vi "Target Resistance.vi"(0 "instrument handle":refnum<k15>="PXI1Slot2 (869)", 1 "Max attempts":dbl=10.0 format="%#_13g", 5 "Lower resistance (ohm)":dbl=80000.0, 9 "Upper resistance (ohm)":dbl=100000.0, 11 "error in (no error)":errorcluster) -> (3 "SL voltage (V)":dbl=2.6, 4 "instrument handle out":refnum<k15>="PXI1Slot2 (869)", 6 "final resistance (ohm)":dbl format="%#_6p", 8 "target hit?":bool, 10 "final current (A)":dbl, 12 "BL voltage (V)":dbl=2.6, 14 "WL voltage (V)":dbl=1.7, 15 "error out":errorcluster)   [LabVIEW 2018]
panel:
  out "attempt number":i32=15
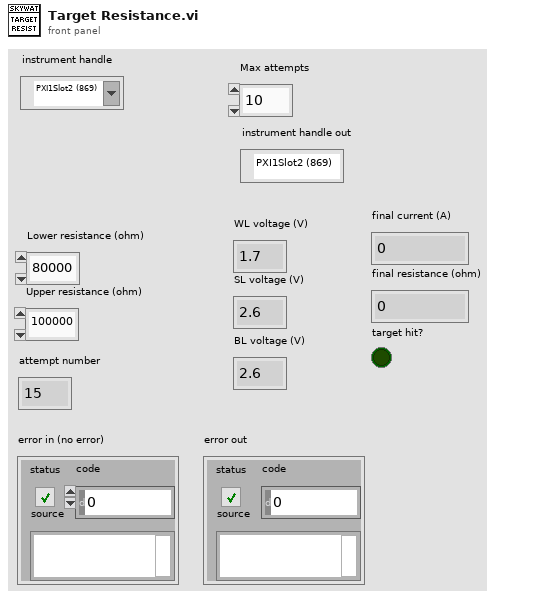
[diagram p1: front panel]
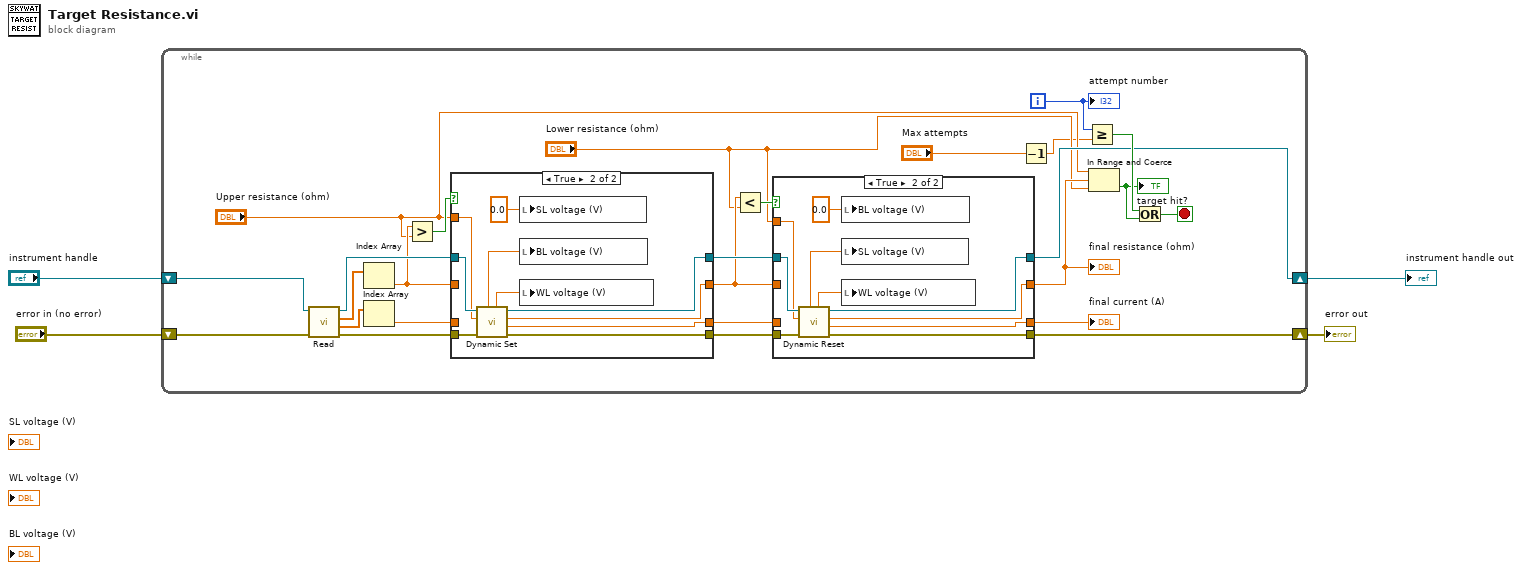
[diagram p0: block diagram]
diagram:
  n1 = while {
    shift-right: [w18] -> w3
    shift-left: "instrument handle" -> [w30]
    shift-right: [w17] -> w2
    shift-left: "error in (no error)" -> [w29]
    i -> [w23]
    stop <- w24 stop-if-true
    n2 = call "Read.vi"("error in (no error)"=w29, "instrument handle"=w30) -> ("error out"=w25:errorcluster, "currents (A)"=w15:dbl[], "resistances (ohm)"=w28:dbl[], "instrument handle out"=w26:refnum<k15>)  [unwired: 6 in]
    n3 = Index Array(array=w28) -> (element=w16:dbl)  [unwired: 1 in]
    n4 = Index Array(array=w15) -> (element=w14:dbl)  [unwired: 1 in]
    n5 = Greater?(x=w16, y="Upper resistance (ohm)") -> (0:w27:bool)
    n6 = case shown="True" w27 {
      tunnel: w26 -> [w48 w56]
      tunnel: w25 -> [w47 w55]
      tunnel: [w48 w57] -> w20
      tunnel: [w47 w58] -> w19
      tunnel: [w46 w54] -> w8
      tunnel: w16 -> [w46 _]
      tunnel: w14 -> [w45 _]
      tunnel: [w45 w53] -> w13
      tunnel: "Upper resistance (ohm)" -> [_ w49]
      frame False {
      }
      frame True {
        n7 = call "Dynamic Set.vi"("error in (no error)"=w55, "target resistance (ohm)"=w49, "instrument handle"=w56) -> ("error out"=w58:errorcluster, "final current (A)"=w53:dbl, "final resistance (ohm)"=w54:dbl, "instrument handle out"=w57:refnum<k15>, "WL voltage (V)"=w52:dbl, "BL voltage (V)"=w51:dbl)  [unwired: 2 in, 1 out]
        n8 = local write "SL voltage (V)"(0.0 ("SL voltage (V)")) -> ()
        n9 = local write "BL voltage (V)"(w51) -> ()
        n10 = local write "WL voltage (V)"(w52) -> ()
      }
    }
    n11 = Less?(x=w8, y="Lower resistance (ohm)") -> (x < y?=w9:bool)
    n12 = case shown="True" w9 {
      tunnel: w20 -> [w34 w42]
      tunnel: w19 -> [w33 w41]
      tunnel: [w34 w43] -> w18
      tunnel: [w33 w44] -> w17
      tunnel: [w32 w40] -> w11
      tunnel: w8 -> [w32 _]
      tunnel: [w31 w39] -> w12
      tunnel: w13 -> [w31 _]
      tunnel: "Lower resistance (ohm)" -> [_ w38]
      frame False {
      }
      frame True {
        n13 = call "Dynamic Reset.vi"("error in (no error)"=w41, "target resistance (ohm)"=w38, "instrument handle"=w42) -> ("error out"=w44:errorcluster, "final current (A)"=w39:dbl, "final resistance (ohm)"=w40:dbl, "instrument handle out"=w43:refnum<k15>, "WL voltage (V)"=w37:dbl, "SL voltage (V)"=w36:dbl)  [unwired: 2 in, 1 out]
        n14 = local write "BL voltage (V)"(0.0 ("BL voltage (V)")) -> ()
        n15 = local write "SL voltage (V)"(w36) -> ()
        n16 = local write "WL voltage (V)"(w37) -> ()
      }
    }
    "final current (A)" <- w12
    "final resistance (ohm)" <- w11
    n17 = Decrement(x="Max attempts") -> (x-1=w5:dbl)
    n18 = Greater Or Equal?(x=w23, y=w5) -> (x >= y?=w22:bool)
    n19 = In Range and Coerce(upper limit="Upper resistance (ohm)", x=w11, lower limit="Lower resistance (ohm)") -> (In Range?=w21:bool)  [unwired: 1 out]
    "target hit?" <- w21
    n20 = Or(x=w22, y=w21) -> (x .or. y?=w24:bool)
    "attempt number" <- w23
  }
  "error out" <- w2
  "instrument handle out" <- w3
